vi "Destructor.vi"(8 "error in":errorcluster, 11 "PID in":refnum<class "INL PID.lvclass">) -> (0 "error out":errorcluster, 3 "PID out":refnum<class "INL PID.lvclass">)   [LabVIEW 2011, in "INL PID.lvclass"]
uses:
  INL PID.lvclass
  INL PID.lvclass/INL PID.ctl
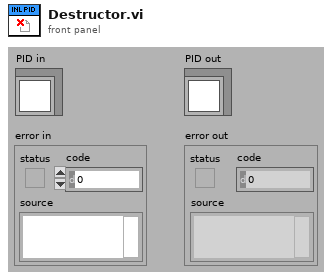
[diagram p1: front panel]
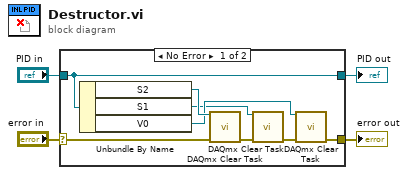
[diagram p0: block diagram]
diagram:
  n1 = case shown="No Error" "error in" {
    selector: "error in" -> [w12 w14]
    tunnel: [w11 w14] -> w3
    tunnel: [w10 w13] -> w1
    tunnel: "PID in" -> [w10 w13]
    frame No Error {
      n2 = Unbundle By Name(w10) -> ("S2"=w8:refnum<k21>, "S1"=w6:refnum<k21>, "V0"=w7:refnum<k21>)
      n3 = call <vilib>:"DAQmx Clear Task.vi"("task in"=w8, "error in"=w12) -> ("error out"=w5:errorcluster)  [unwired: 13 in]
      n4 = call <vilib>:"DAQmx Clear Task.vi"("task in"=w6, "error in"=w5) -> ("error out"=w9:errorcluster)  [unwired: 13 in]
      n5 = call <vilib>:"DAQmx Clear Task.vi"("task in"=w7, "error in"=w9) -> ("error out"=w11:errorcluster)  [unwired: 13 in]
    }
    frame Error {
    }
  }
  "error out" <- w3
  "PID out" <- w1
